vi "pass_pipe.vi"(7 "bird":sgl, 8 "error in (no error)":errorcluster, 9 "y lower":sgl, 10 "y upper":sgl, 11 "Start?":bool) -> (0 "error out":errorcluster, 2 "pass":bool)   [LabVIEW 2017, in "Flappy Bird.lvlib"]
uses:
  Flappy Bird.lvlib
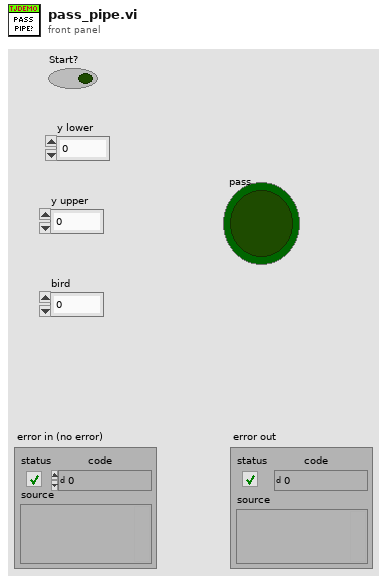
[diagram p1: front panel]
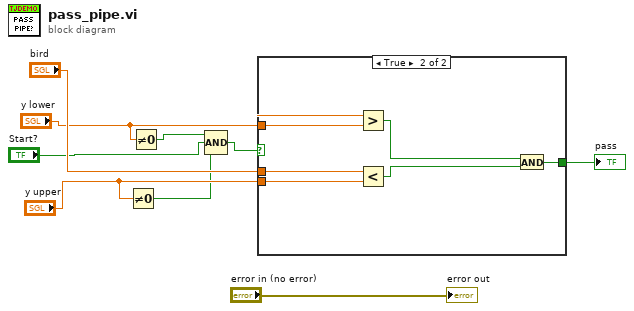
[diagram p0: block diagram]
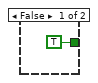
[diagram p2: hidden frame]
diagram:
  n1 = Not Equal To 0?(x="y upper") -> (x != 0?=w4:bool)
  n2 = Not Equal To 0?(x="y lower") -> (x != 0?=w2:bool)
  n3 = Compound Arithmetic op=AND(w2, "Start?", w4) -> (w1:bool)
  n4 = case shown="True" w1 {
    tunnel: [TRUE w14] -> w8
    tunnel: "bird" -> [_ w13]
    tunnel: "y lower" -> [_ w12]
    tunnel: "y upper" -> [_ w11]
    frame False {
    }
    frame True {
      n5 = Greater?(x=w13, y=w12) -> (0:w16:bool)
      n6 = Less?(x=w13, y=w11) -> (x < y?=w15:bool)
      n7 = And(x=w16, y=w15) -> (x .and. y?=w14:bool)
    }
  }
  "pass" <- w8
  "error out" <- "error in (no error)"
